vi "b2g2_sqlite_write_time.vi"(8 "error in (no error)":errorcluster, 9 "output cluster timestamp":timestamp, 10 "Database File":string, 11 "Output - Cluster b2g1":T1 {"TS-5 [°C]" format="%#.2g"; "pHS-1 [pH]" format="%.2g"; "TS-4 [°C]" format="%#.2g"; "FS-2 [l]" format="%.2g"; "FS-1 [l]" format="%.2g"; "DS-1 [bar]" format="%#.2g"; "DFS-1 [l/min]" format="%#.2g"; "FS-3 [l]" format="%.2g"; "DFS-1 [dl]" format="%.0g"}) -> (0 "error out":errorcluster)   [LabVIEW 2011]
uses:
  Output - Cluster b2g2.ctl
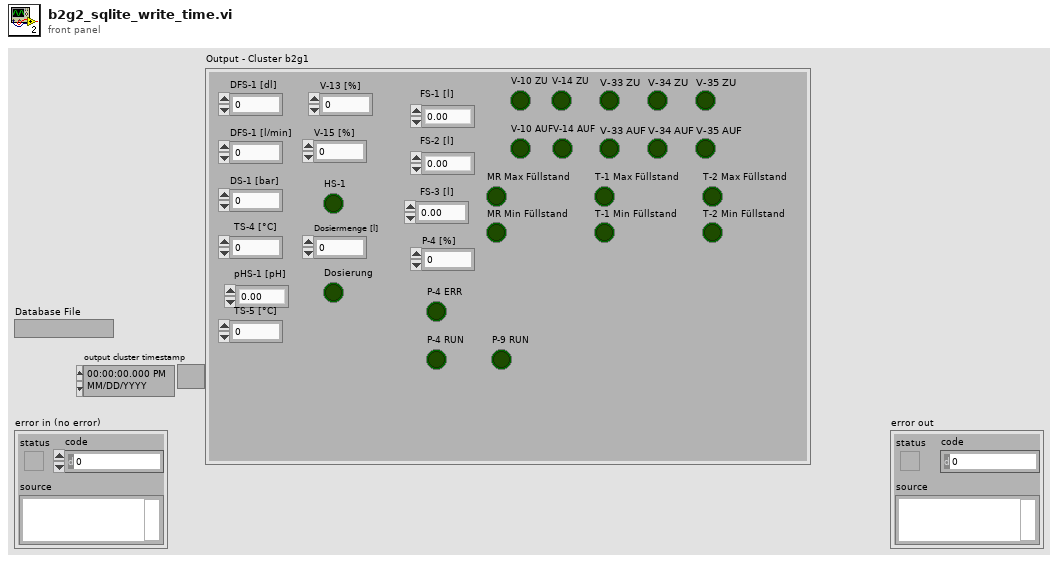
[diagram p1: front panel]
types:
  T1 = typedef "Output - Cluster b2g2.ctl" = cluster{"DFS-1 [dl]":u64, "FS-3 [l]":dbl, "DFS-1 [l/min]":dbl, "DS-1 [bar]":dbl, "V-10 ZU":bool, "V-14 ZU":bool, "FS-1 [l]":dbl, "FS-2 [l]":dbl, "TS-4 [°C]":dbl, "HS-1":bool, "V-13 [%]":u8, "V-15 [%]":u8, "P-4 [%]":u8, "Dosierung":bool, "MR Max Füllstand":bool, "MR Min Füllstand":bool, "Dosiermenge [l]":sgl, "V-14 AUF":bool, "V-10 AUF":bool, "T-1 Max Füllstand":bool, "T-1 Min Füllstand":bool, "T-2 Max Füllstand":bool, "T-2 Min Füllstand":bool, "pHS-1 [pH]":dbl, "P-4 RUN":bool, "V-33 AUF":bool, "V-33 ZU":bool, "V-34 AUF":bool, "V-34 ZU":bool, "P-4 ERR":bool, "TS-5 [°C]":dbl, "V-35 AUF":bool, "V-35 ZU":bool, "P-9 RUN":bool}
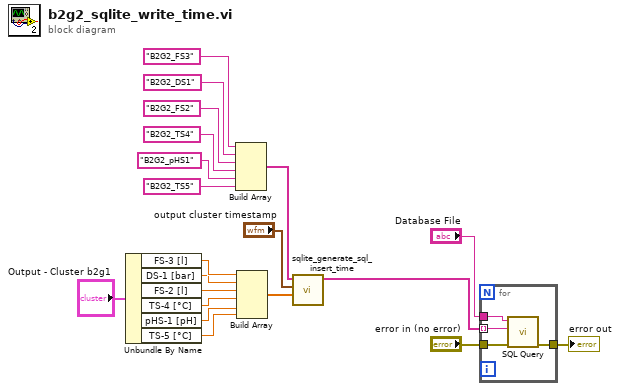
[diagram p0: block diagram]
diagram:
  n1 = Unbundle By Name("Output - Cluster b2g1") -> ("FS-3 [l]"=w20:dbl, "DS-1 [bar]"=w19:dbl, "FS-2 [l]"=w18:dbl, "TS-4 [°C]"=w17:dbl, "pHS-1 [pH]"=w16:dbl, "TS-5 [°C]"=w15:dbl)
  n2 = Build Array("B2G2_FS3" ("SQL Query"), "B2G2_DS1" ("SQL Query"), "B2G2_FS2" ("SQL Query"), "B2G2_TS4" ("SQL Query"), "B2G2_pHS1" ("SQL Query"), "B2G2_TS5" ("SQL Query")) -> (w8:string[])
  n3 = Build Array(w20, w19, w18, w17, w16, w15) -> (w7:dbl[])
  n4 = call "sqlite_generate_sql_insert_time.vi"("Array"=w7, "output cluster timestamp"="output cluster timestamp", "Array 2"=w8) -> ("Array 3"=w5:string[])  [unwired: 8 in]
  n5 = for {
    tunnel: "Database File" -> [w24]
    tunnel: w5 -> [w23] mode=indexing
    tunnel: "error in (no error)" -> [w22]
    tunnel: [w21] -> w3
    n6 = call "SQL Query.vi"("error in (no error)"=w22, "SQL Query"=w23, "Database File"=w24) -> ("error out"=w21:errorcluster)  [unwired: 6 in, 2 out]
  }
  "error out" <- w3
